vi "Analyze_Splitting_vs_Angle.vi"(11 "X,Y,Z1, Z2, ...":dbl[][](array[numeric])=array2435x8[19480 elements]) -> (3 "Intensity Graph":dbl[][](graph))   [LabVIEW 2016]
uses:
  <vilib>/gmath/NumericalOptimization/Nonlinear Curve Fit LM formula string.vi
  <vilib>/gmath/NI_Gmath.lvlib
  <vilib>/Analysis/NI_AALPro.lvlib
panel:
  out "best fit parameters 2":dbl[](array[numeric])=[10.0, 160.0, 170.0]
  in  "initial parameters 2":dbl[](array[numeric])=[10.0, 160.0, 170.0]
  in  "model description 2":T1={"model"="a*sin(3.14/180*(x-b))+c", "Parameters"=["a", "b", "c"], "x"="x"}
  in  "which fitting parameter to plot":i32=1
  in  "Enum 2":enum16{"All Phi", "Phi from cursor"}(ring)=enum."Phi from cursor"
  in  "Load New Data?":bool
  in  "STOP":bool=TRUE
  in  "2D Array Settings":T2={"x Max"=270.0, "x Min"=65.0, "x step size"=2.5, "y Max"=320.0, "y Min"=5.0, "y step size"=2.5} {"y step size" format="%#_13g"; "y Min" format="%#_13g"; "y Max" format="%#_13g"; "x step size" format="%#_13g"; "x Min" format="%#_13g"; "x Max" format="%#_13g"}
  in  "limits 2":T3={"X upper limit"=260.0, "X lower limit"=60.0, "Y upper limit"=180.0, "Y lower limit"=0.0} {"Y lower limit" format="%#_13g"; "Y upper limit" format="%#_13g"; "X lower limit" format="%#_13g"; "X upper limit" format="%#_13g"}
  in  "limits":T3={"X upper limit"=215.0, "X lower limit"=120.0, "Y upper limit"=60.0, "Y lower limit"=0.0} {"Y lower limit" format="%#_13g"; "Y upper limit" format="%#_13g"; "X lower limit" format="%#_13g"; "X upper limit" format="%#_13g"}
  in  "String":string="a-((x - b)/c)*((x - b)/c)\n\na*cos(c*(x-b))"
  out "XY Graph 5":cluster{dbl[], "Best Linear Fit":dbl[]}[](graph)=[{[5.0, 7.5, 10.0, 12.5, 15.0, 17.5, 20.0, 22.5, 25.0, 27.5, 30.0, 32.5, 35.0, 37.5, 40.0, 42.5, 45.0, 47.5, 50.0, 52.5, 55.0, 57.5, 60.0, 62.5, 65.0, 67.5, 70.0, 72.5, 75.0, 77.5, 80.0, 82.5, 85.0, 87.5, 90.0, 92.5, 95.0, 97.5, 100.0, 102.5, 105.0, 107.5, 110.0, 112.5, 115.0, 117.5, 120.0, 122.5, 125.0, 127.5, 130.0, 132.5, 135.0, 137.5, 140.0, 142.5, 145.0, 147.5, 150.0, 152.5, 155.0, 157.5, 160.0, 162.5, 165.0, 167.5, 170.0, 172.5, 175.0, 177.5, 180.0, 182.5, 185.0, 187.5, 190.0, 192.5, 195.0, 197.5, 200.0, 202.5, 205.0, 207.5, 210.0, 212.5, 215.0, 217.5, 220.0, 222.5, 225.0, 227.5, 230.0, 232.5, 235.0, 237.5, 240.0, 242.5, 245.0, 247.5, 250.0, 252.5, 255.0, 257.5, 260.0, 262.5, 265.0, 267.5, 270.0, 272.5, 275.0, 277.5, 280.0, 282.5, 285.0, 287.5, 290.0, 292.5, 295.0, 297.5, 300.0, 302.5, 305.0, 307.5, 310.0, 312.5, 315.0, 317.5, 320.0], "Best Linear Fit"=[158.21586008274636]}, {[5.0, 7.5, 10.0, 12.5, 15.0, 17.5, 20.0, 22.5, 25.0, 27.5, 30.0, 32.5, 35.0, 37.5, 40.0, 42.5, 45.0, 47.5, 50.0, 52.5, 55.0, 57.5, 60.0, 62.5, 65.0, 67.5, 70.0, 72.5, 75.0, 77.5, 80.0, 82.5, 85.0, 87.5, 90.0, 92.5, 95.0, 97.5, 100.0, 102.5, 105.0, 107.5, 110.0, 112.5, 115.0, 117.5, 120.0, 122.5, 125.0, 127.5, 130.0, 132.5, 135.0, 137.5, 140.0, 142.5, 145.0, 147.5, 150.0, 152.5, 155.0, 157.5, 160.0, 162.5, 165.0, 167.5, 170.0, 172.5, 175.0, 177.5, 180.0, 182.5, 185.0, 187.5, 190.0, 192.5, 195.0, 197.5, 200.0, 202.5, 205.0, 207.5, 210.0, 212.5, 215.0, 217.5, 220.0, 222.5, 225.0, 227.5, 230.0, 232.5, 235.0, 237.5, 240.0, 242.5, 245.0, 247.5, 250.0, 252.5, 255.0, 257.5, 260.0, 262.5, 265.0, 267.5, 270.0, 272.5, 275.0, 277.5, 280.0, 282.5, 285.0, 287.5, 290.0, 292.5, 295.0, 297.5, 300.0, 302.5, 305.0, 307.5, 310.0, 312.5, 315.0, 317.5, 320.0], "Best Linear Fit"=[0.0, 0.0, 0.0, 0.0, 0.0, 0.0, 0.0, 0.0, 0.0, 0.0, 0.0, 0.0, 0.0, 0.0, 0.0, 0.0, 0.0, 0.0, 0.0, 0.0, 0.0, 0.0, 0.0, 0.0, 0.0, 0.0, 0.0, 0.0, 0.0, 0.0, 0.0, 0.0, 0.0, 0.0, 0.0, 0.0, 0.0, 0.0, 0.0, 0.0, 0.0, 0.0, 0.0, 0.0, 0.0, 0.0, 0.0, 0.0, 0.0, 0.0, 0.0, 0.0, 0.0, 0.0, 0.0, 0.0, 0.0, 0.0, 0.0, 0.0, 0.0, 0.0, 0.0, 0.0, 0.0, 0.0, 0.0, 0.0, 0.0, 0.0, 0.0, 0.0, 0.0, 0.0, 0.0, 0.0, 0.0, 0.0, 0.0, 0.0, 0.0, 0.0, 0.0, 0.0, 0.0, 0.0, 0.0, 0.0, 0.0, 0.0, 0.0, 0.0, 0.0, 0.0, 0.0, 0.0, 0.0, 0.0, 0.0, 0.0, 0.0, 0.0, 0.0, 0.0, 0.0, 0.0, 0.0, 0.0, 0.0, 0.0, 0.0, 0.0, 0.0, 0.0, 0.0, 0.0, 0.0, 0.0, 0.0, 0.0, 0.0, 0.0, 0.0, 0.0, 0.0, 0.0, 0.0]}]
  out "best fit parameters":dbl[](array[numeric])=[50.324461350377526, 158.21586008274636, -25.837217688532053]
  in  "initial parameters":dbl[](array[numeric])=[10.0, 170.0, 10.0]
  in  "model description":T1={"model"="a*cos(3.14/180*(x-b))*cos(3.14/180*(x-b))+c", "Parameters"=["a", "b", "c"], "x"="x"}
  in  "Enum":T4(ring)
  out "XY Graph 4":cluster{"Waveform Graph":dbl[], dbl[]}[](graph)=[{"Waveform Graph"=[65.0, 67.5, 70.0, 72.5, 75.0, 77.5, 80.0, 82.5, 85.0, 87.5, 90.0, 92.5, 95.0, 97.5, 100.0, 102.5, 105.0, 107.5, 110.0, 112.5, 115.0, 117.5, 120.0, 122.5, 125.0, 127.5, 130.0, 132.5, 135.0, 137.5, 140.0, 142.5, 145.0, 147.5, 150.0, 152.5, 155.0, 157.5, 160.0, 162.5, 165.0, 167.5, 170.0, 172.5, 175.0, 177.5, 180.0, 182.5, 185.0, 187.5, 190.0, 192.5, 195.0, 197.5, 200.0, 202.5, 205.0, 207.5, 210.0, 212.5, 215.0, 217.5, 220.0, 222.5, 225.0, 227.5, 230.0, 232.5, 235.0, 237.5, 240.0, 242.5, 245.0, 247.5, 250.0, 252.5, 255.0, 257.5, 260.0, 262.5, 265.0, 267.5, 270.0], [-1.0, -1.0, -1.0, -1.0, -1.0, -1.0, -1.0, -1.0, -1.0, -1.0, -1.0, -1.0, -1.0, -1.0, -1.0, -1.0, -1.0, -1.0, -1.0, -1.0, -1.0, -1.0, -1.0, -1.0, -1.0, -1.0, -1.0, -1.0, -1.0, 18.418380709944255, 19.535911391444284, 20.466898621255627, 21.78744699669355, 22.5401738211584, 23.818559390972425, 24.547534188555957, 23.841433300349628, -1.0, -1.0, -1.0, -1.0, -1.0, -1.0, -1.0, -1.0, -1.0, -1.0, -1.0, -1.0, -1.0, -1.0, -1.0, -1.0, -1.0, -1.0, -1.0, -1.0, -1.0, -1.0, -1.0, -1.0, -1.0, -1.0, -1.0, -1.0, -1.0, -1.0, -1.0, -1.0, -1.0, -1.0, -1.0, -1.0, -1.0, -1.0, -1.0, -1.0, -1.0, -1.0, -1.0, -1.0, -1.0]}, {"Waveform Graph"=[65.0, 67.5, 70.0, 72.5, 75.0, 77.5, 80.0, 82.5, 85.0, 87.5, 90.0, 92.5, 95.0, 97.5, 100.0, 102.5, 105.0, 107.5, 110.0, 112.5, 115.0, 117.5, 120.0, 122.5, 125.0, 127.5, 130.0, 132.5, 135.0, 137.5, 140.0, 142.5, 145.0, 147.5, 150.0, 152.5, 155.0, 157.5, 160.0, 162.5, 165.0, 167.5, 170.0, 172.5, 175.0, 177.5, 180.0, 182.5, 185.0, 187.5, 190.0, 192.5, 195.0, 197.5, 200.0, 202.5, 205.0, 207.5, 210.0, 212.5, 215.0, 217.5, 220.0, 222.5, 225.0, 227.5, 230.0, 232.5, 235.0, 237.5, 240.0, 242.5, 245.0, 247.5, 250.0, 252.5, 255.0, 257.5, 260.0, 262.5, 265.0, 267.5, 270.0], [-25.683463517298065, -25.830339145701984, -25.785961294277126, -25.550667363130934, -25.126246267118493, -24.5159248349122, -23.724343275764923, -22.757519900490145, -21.62280536488183, -20.328826783456435, -18.8854221384143, -17.303565482502236, -15.59528350445201, -13.773564091338768, -11.852257583050275, -9.845971469618654, -7.76995933201971, -5.640004870811225, -3.472301904328134, -1.283331248795708, 0.910264583571923, 3.0918079158306853, 5.24471270491917, 7.3526106435886085, 9.399475606910503, 11.369745497208147, 13.24844056103829, 15.02127727867104, 16.67477696017865, 18.19636822248845, 19.57448256827774, 20.798642340034664, 21.85954038057915, 22.74911079439403, 23.460590271774894, 23.988569509557944, 24.329034337479445, 24.479396237487375, 24.438512023970258, 24.206692535276257, 23.78570027044226, 23.178735989100087, 22.390414376439924, 21.426728958247143, 20.295006532760123, 19.00385146579877, 17.563080272681777, 15.983646984299707, 14.277559864777476, 12.457790113913145, 10.53817324851875, 8.533303912450325, 6.458424915075337, 4.3293113418063705, 2.1621506177963603, -0.026580563341561003, -2.2202415100917356, -4.402154050452324, -6.55572933431181, -8.664593956720644, -10.712714443156154, -12.684519150332303, -14.565016655755544, -16.33990973592333, -17.995704066601217, -19.51981081874172, -20.90064237001925, -22.12770040429616, -23.191655729209227, -24.084419205031793, -24.799203245546956, -25.330573423347154, -25.674489787210614, -25.828337577422865, -25.790947105518118, -25.562602647296874, -25.145040281507086, -24.54143469062121, -23.756375024061345, -22.795830007381902, -21.667102562680963, -20.378774285256476, -18.940640198645482]}]
  # "Fit stuff vs theta"
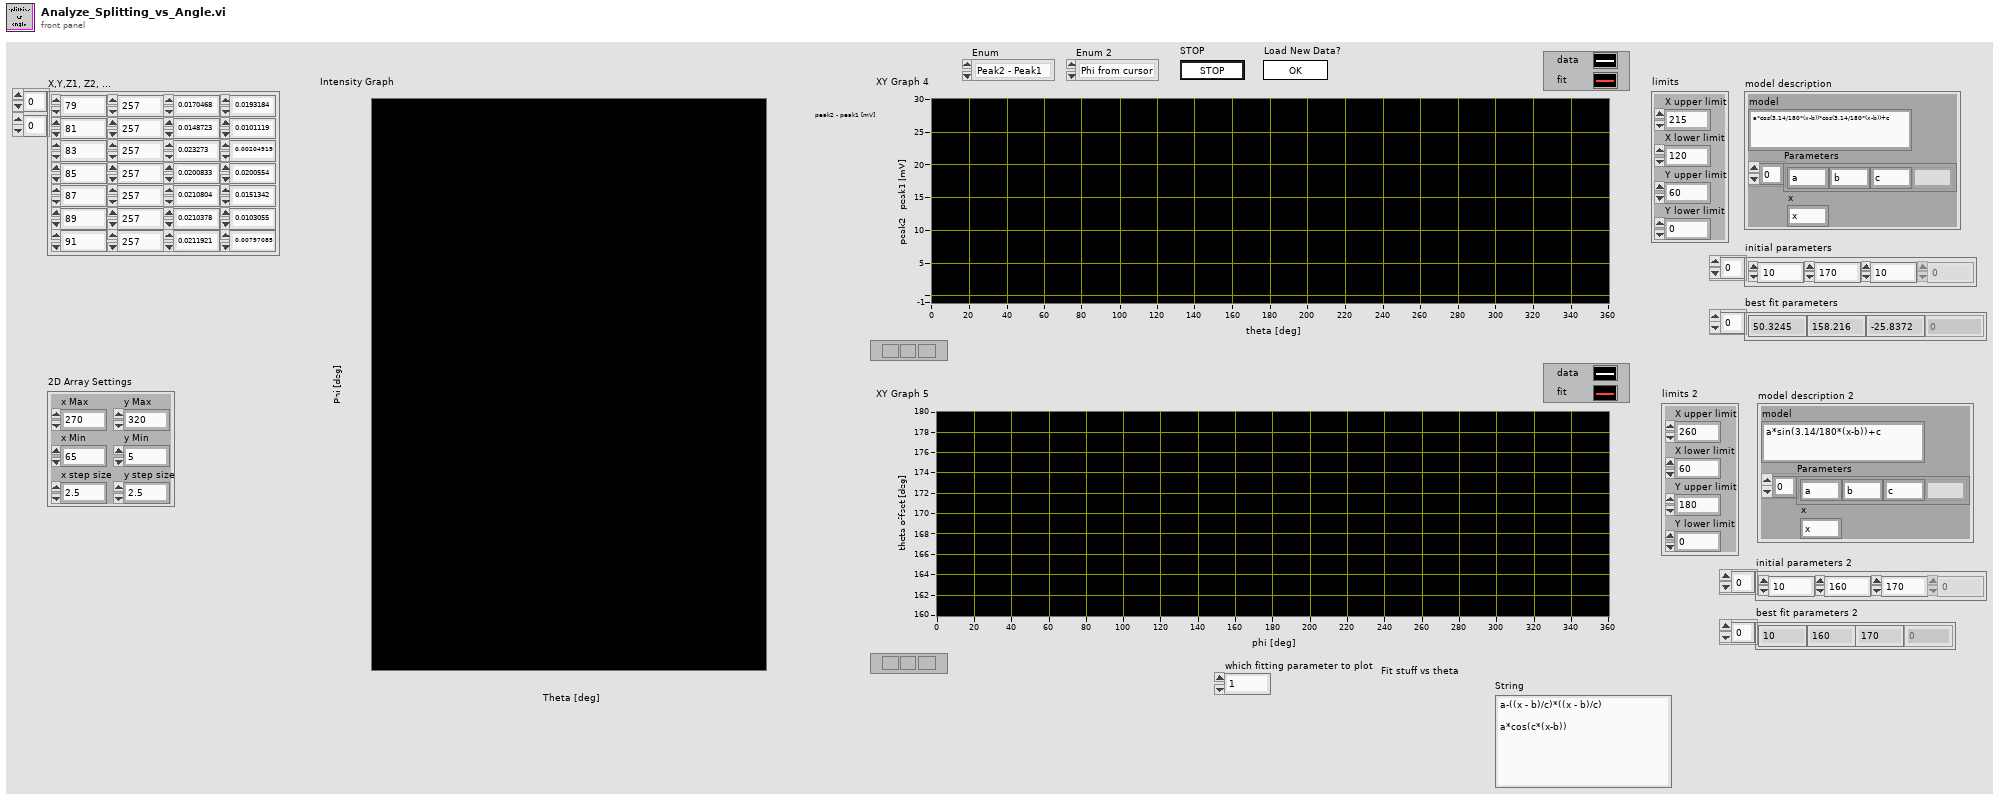
[diagram p1: front panel]
types:
  T1 = cluster{"model":string, "Parameters":string[], "x":string}
  T2 = cluster{"x Max":dbl, "x Min":dbl, "x step size":dbl, "y Max":dbl, "y Min":dbl, "y step size":dbl}
  T3 = cluster{"X upper limit":dbl, "X lower limit":dbl, "Y upper limit":dbl, "Y lower limit":dbl}
  T4 = enum16{"Peak2 - Peak1", "Peak3 - Peak2", "Peak3 - Peak1"}
  T5 = enum32{"invalid app kind", "Development System", "Run Time System", "Student Edition", "Embedded LabVIEW", "Evaluation", "Custom"}
  T6 = enum32{"Invalid", "Standard", "Closed", "Hidden", "Minimized", "Maximized"}
  T7 = cluster{"Core":cluster{"Current VI Reference":refnum<vi>, "Close Panel on Exit?":bool}, "Your Boolean data":bool, "Your string data":string, "2D array":dbl[][], "x array":dbl[], "y array":dbl[], "best fitting":dbl[][], "fitting goodness":dbl[][]}
  T8 = cluster{"Current VI Reference":refnum<vi>, "Close Panel on Exit?":bool}
  T9 = typedef "LVOffsetAndMultiplierTypeDef.ctl" = cluster{"Offset":dbl, "Multiplier":dbl}
  T10 = typedef "LVPointDoubleTypeDef.ctl" = cluster{"Cursor X":dbl, "Cursor Y":dbl}
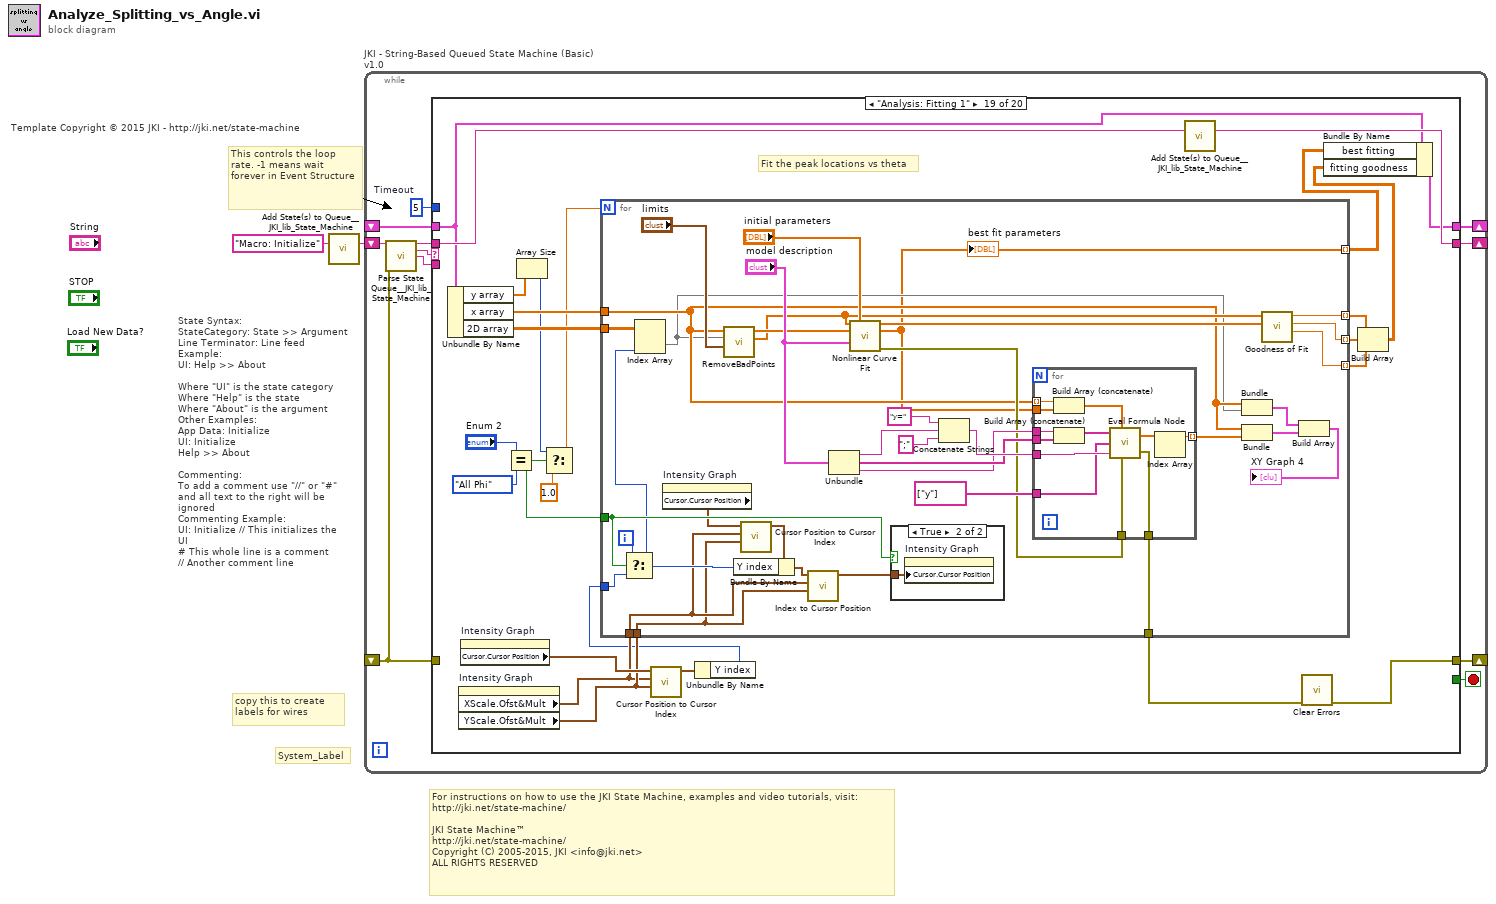
[diagram p0: block diagram]
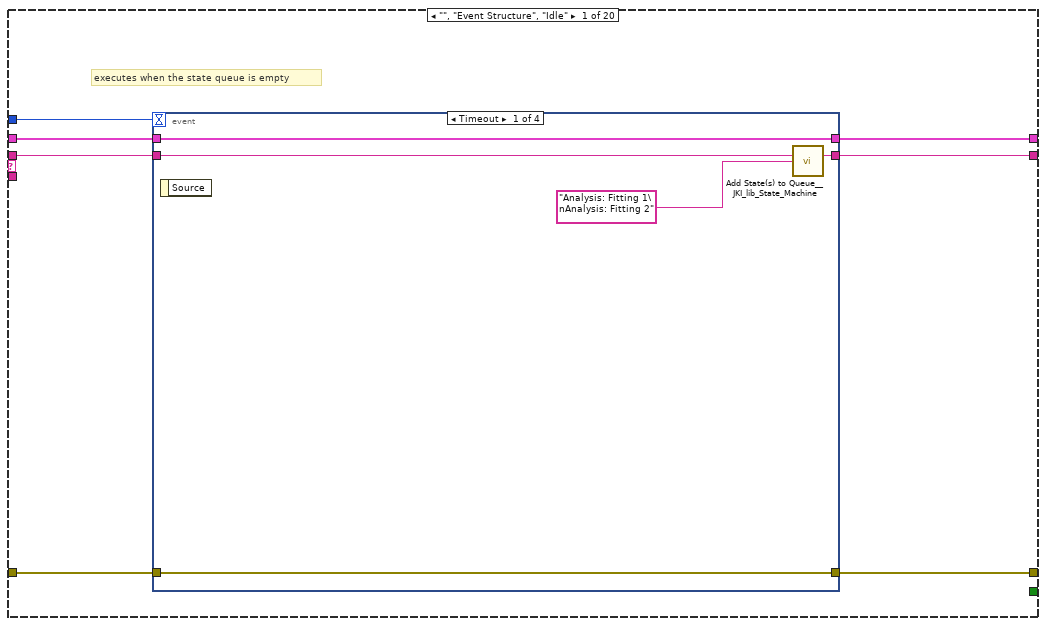
[diagram p2: hidden frame]
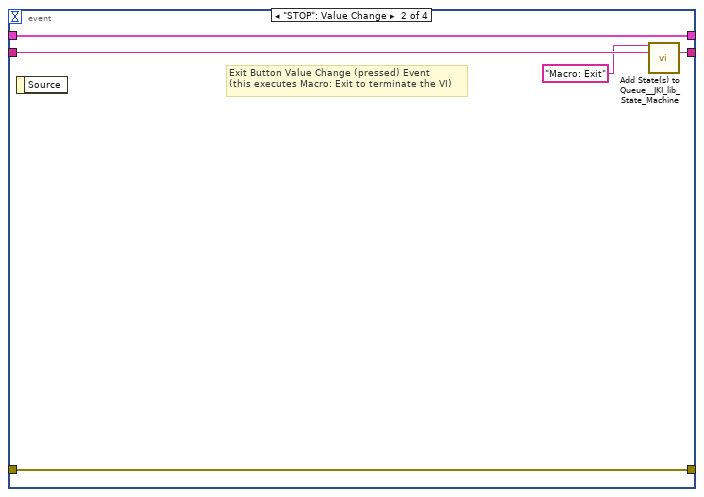
[diagram p3: hidden frame]
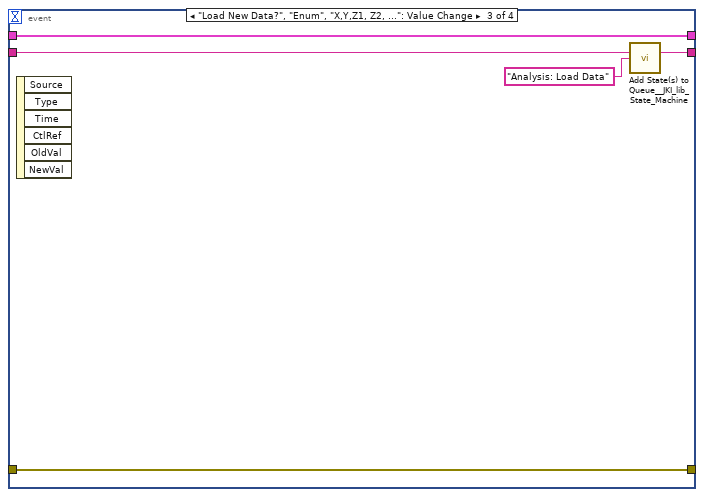
[diagram p4: hidden frame]
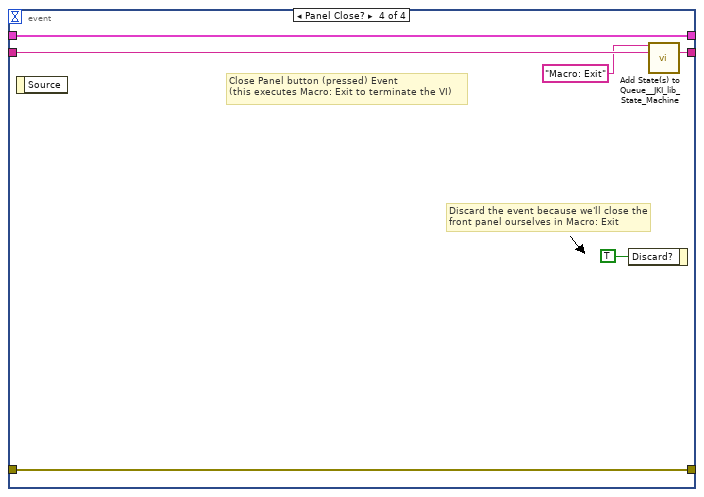
[diagram p5: hidden frame]
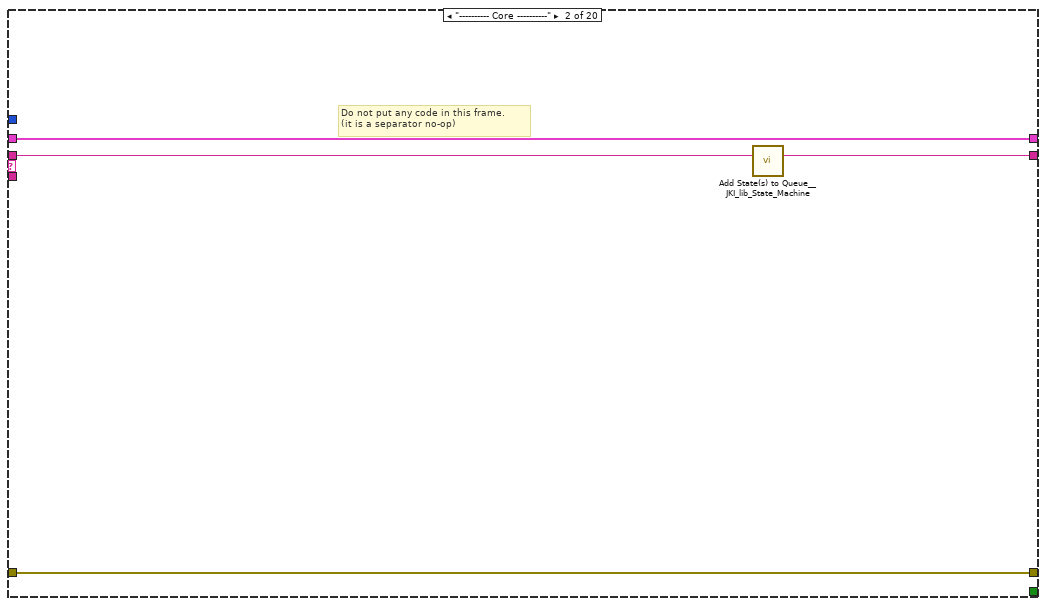
[diagram p6: hidden frame]
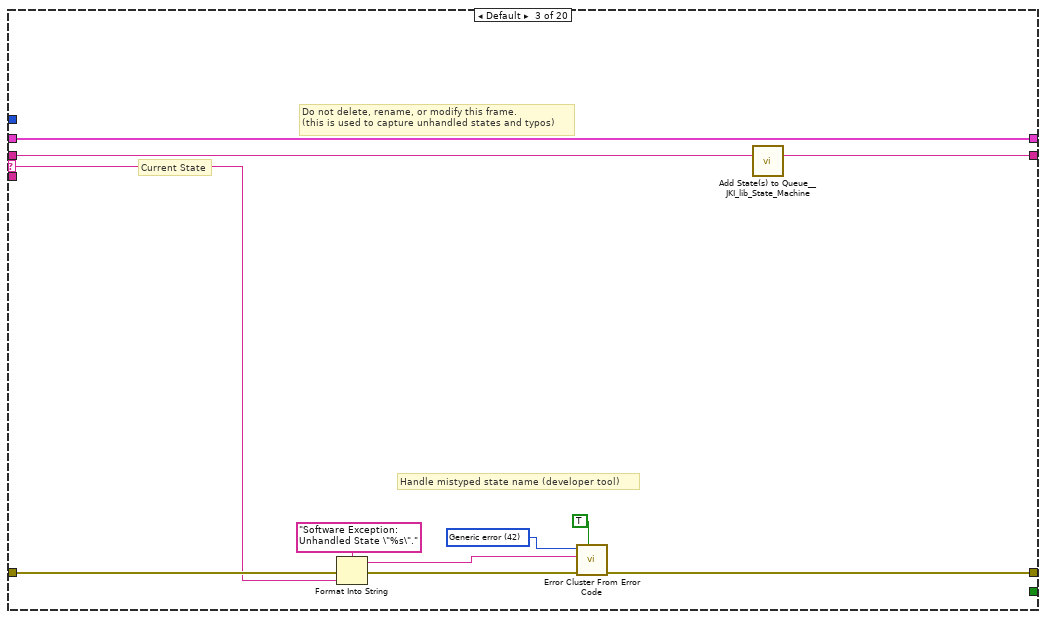
[diagram p7: hidden frame]
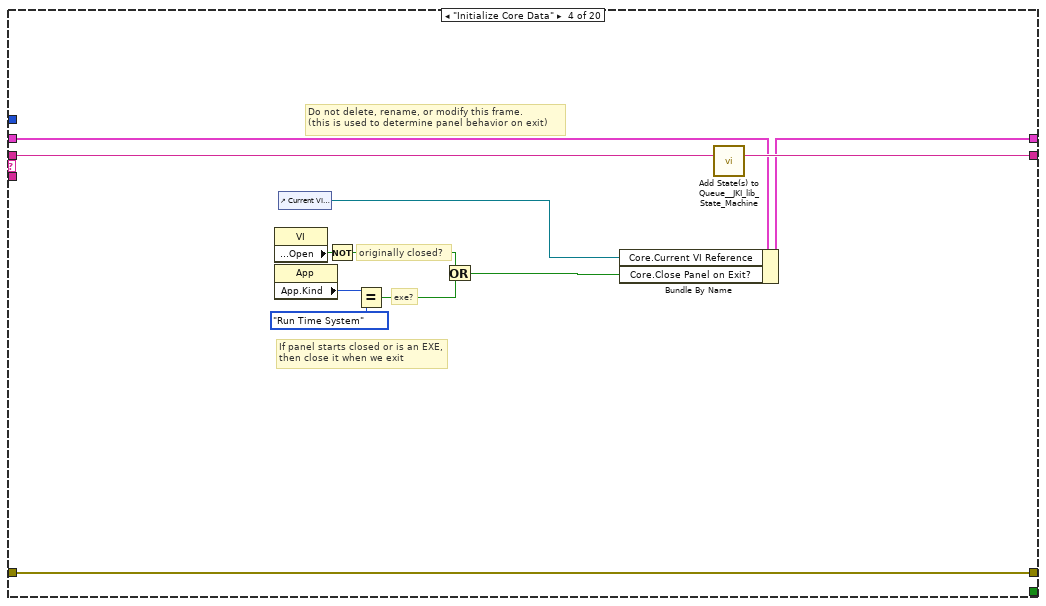
[diagram p8: hidden frame]
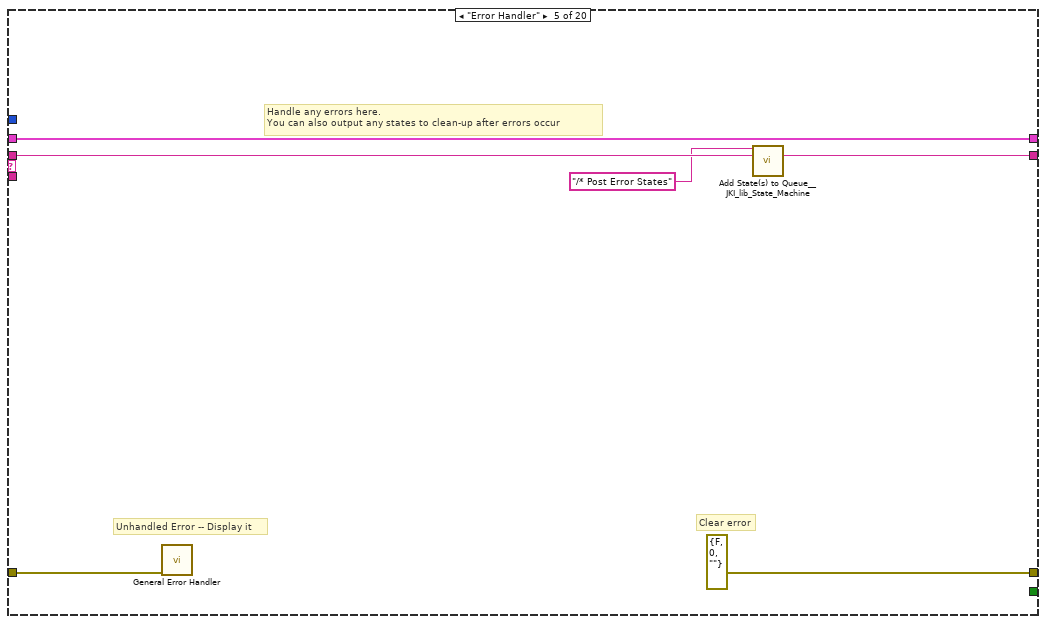
[diagram p9: hidden frame]
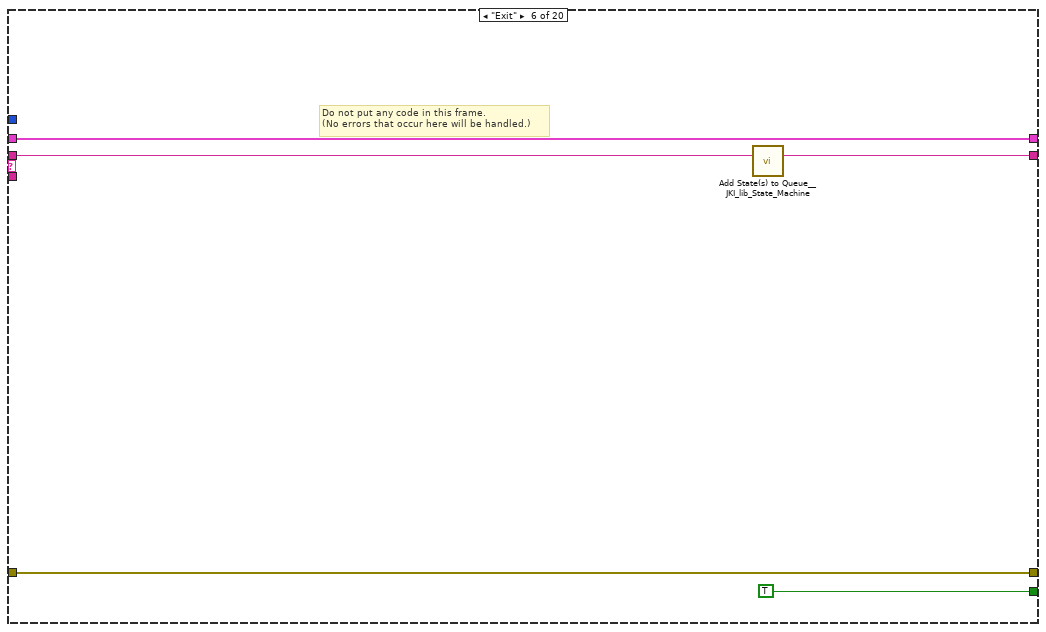
[diagram p10: hidden frame]
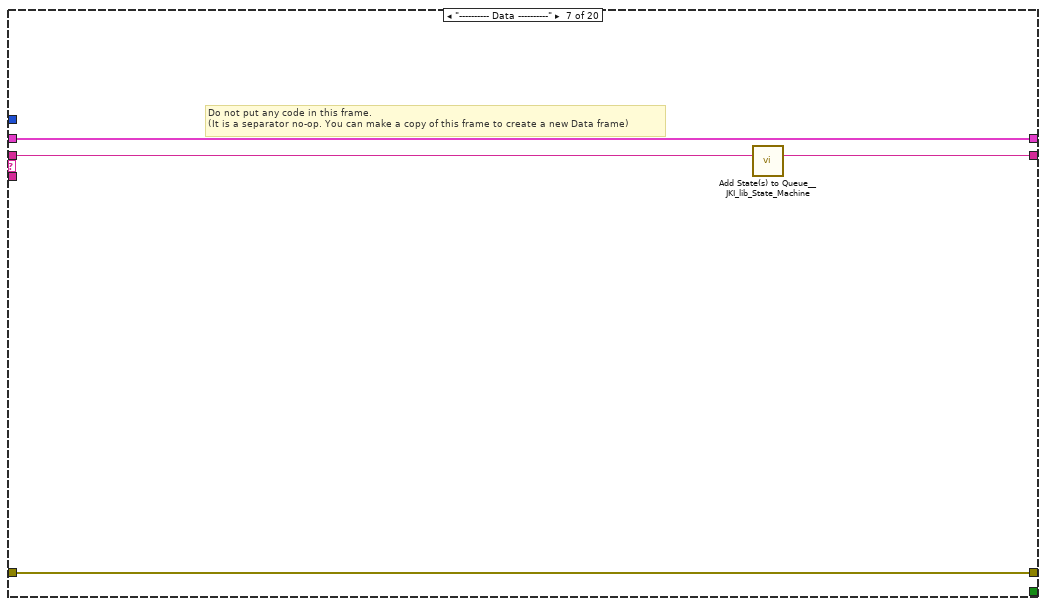
[diagram p11: hidden frame]
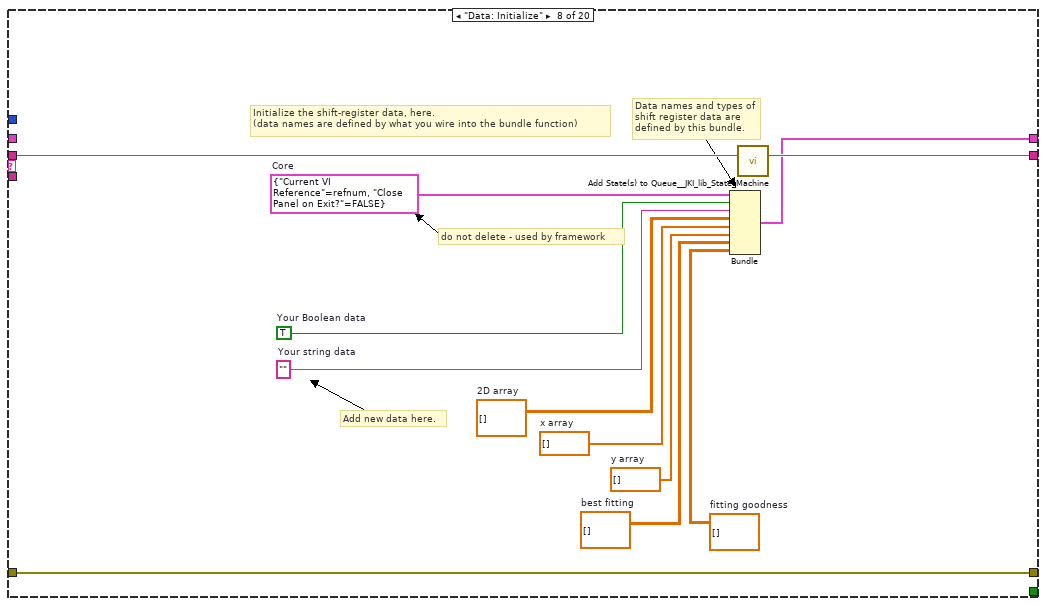
[diagram p12: hidden frame]
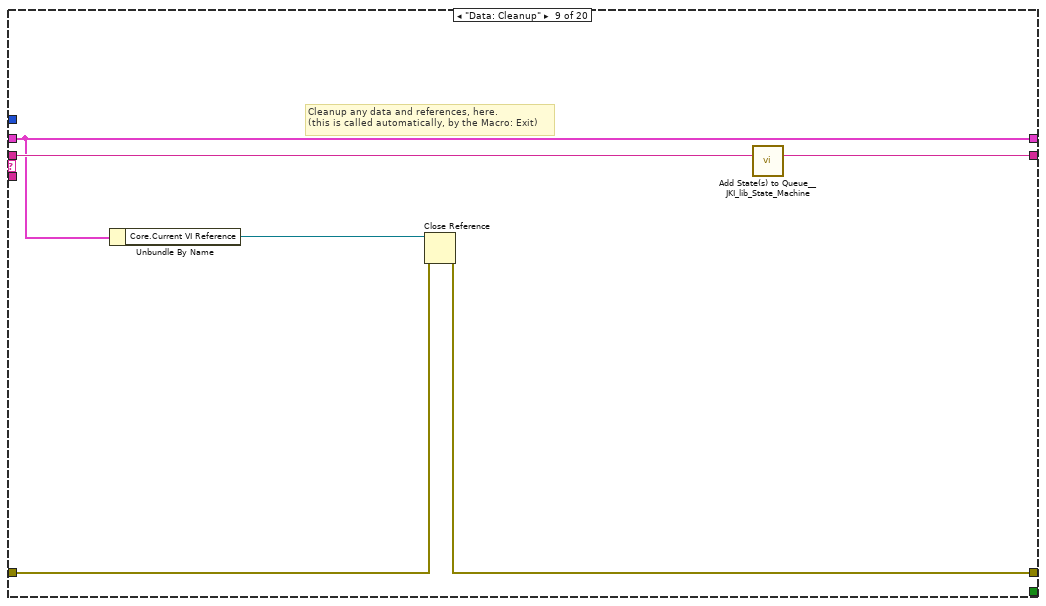
[diagram p13: hidden frame]
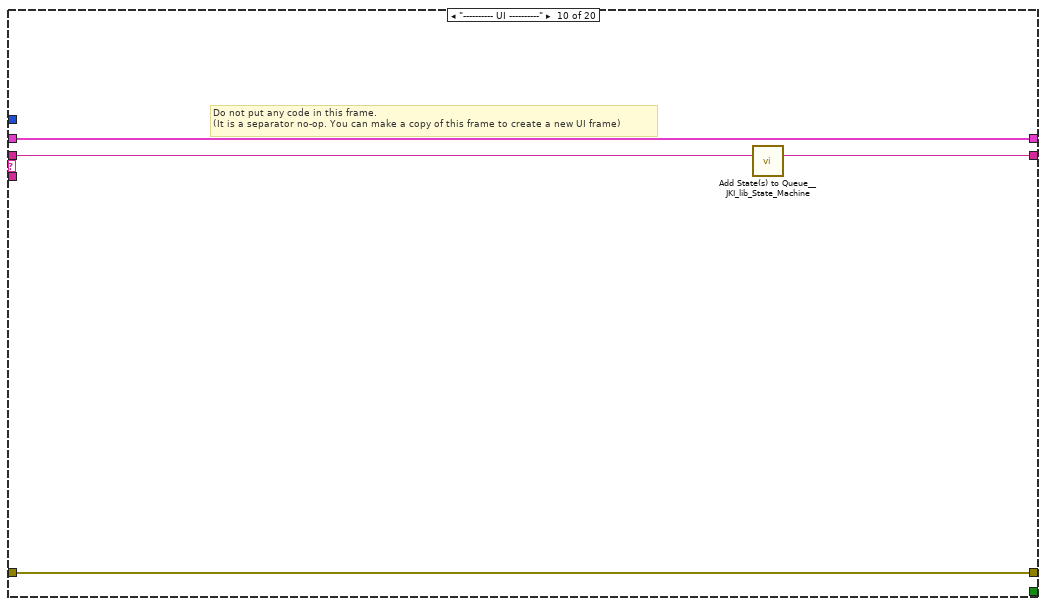
[diagram p14: hidden frame]
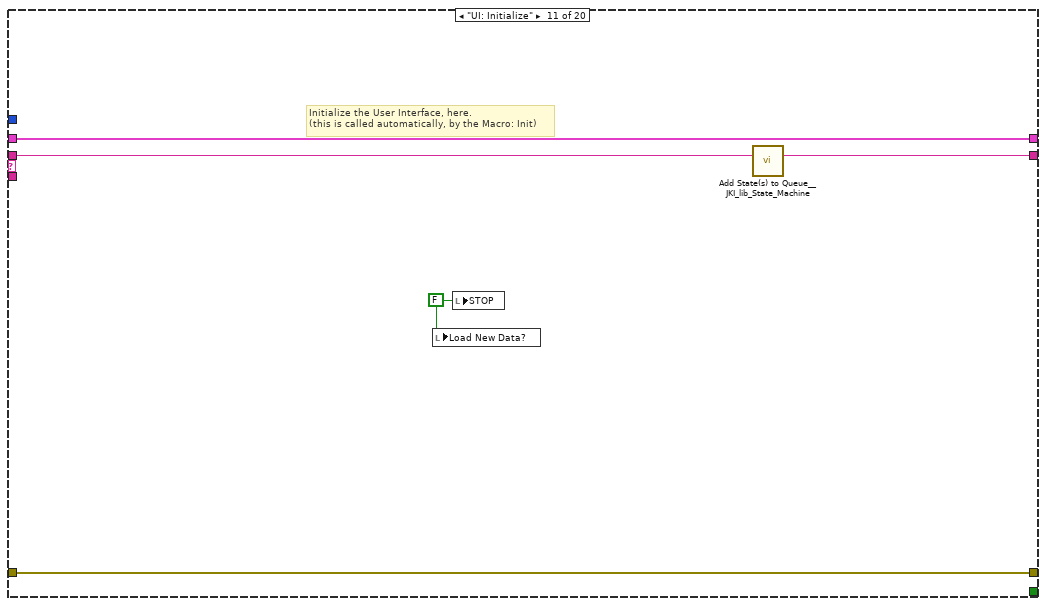
[diagram p15: hidden frame]
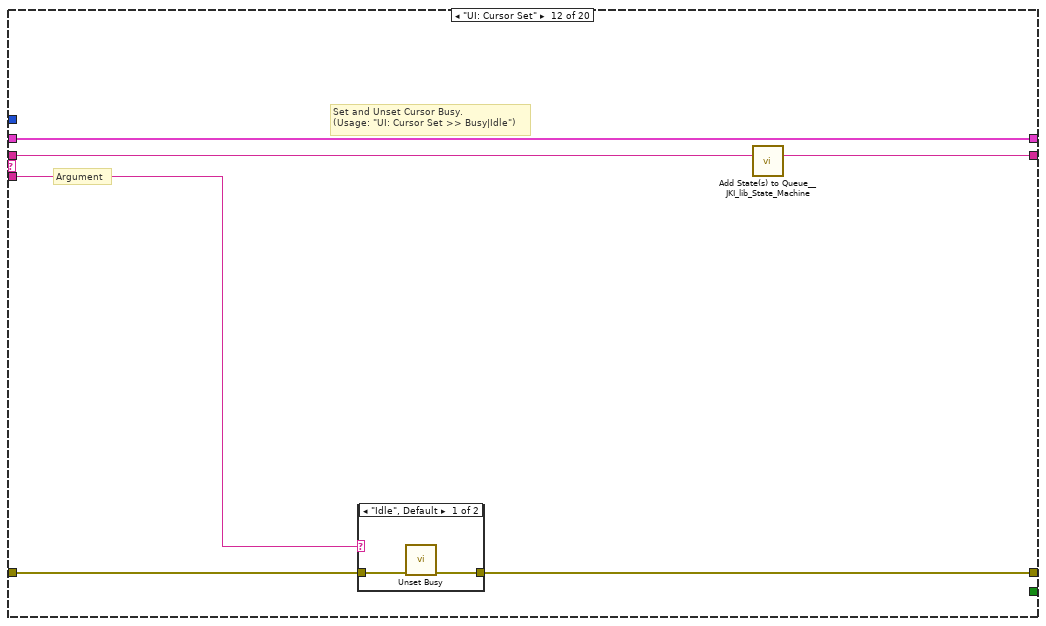
[diagram p16: hidden frame]
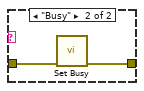
[diagram p17: hidden frame]
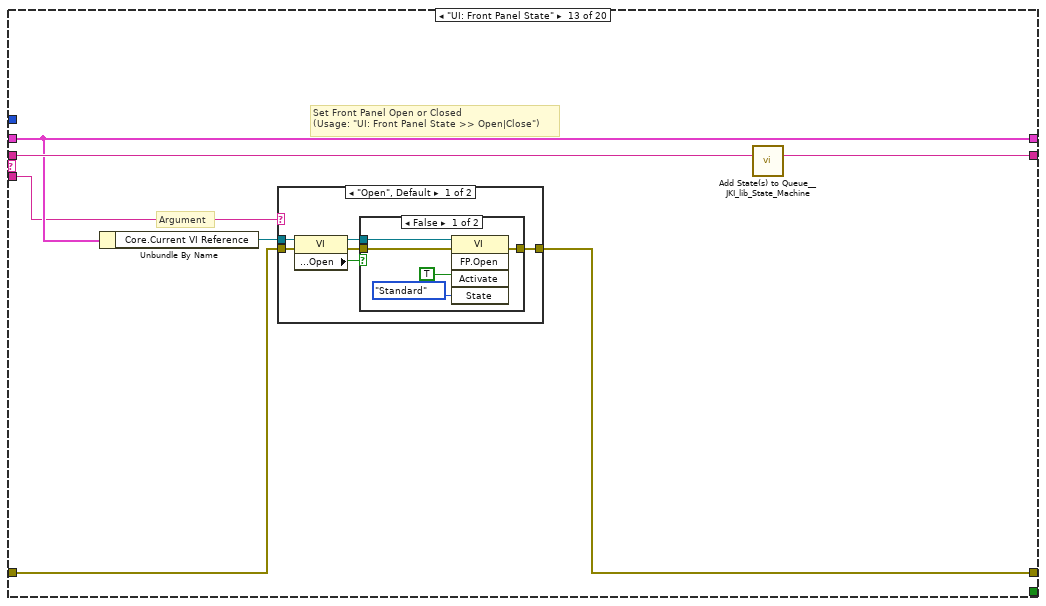
[diagram p18: hidden frame]
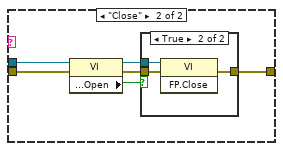
[diagram p20: hidden frame]
diagram:
  # "Template Copyright © 2015 JKI - http://jki.net/state-machine"
  # "For instructions on how to use the JKI State Machine, examples and video tutorials, visit:\nhttp://jki.net/state-machine/\n\nJKI State Machine™\nhttp://jki.net/state-machine/\nCopyright (C) 2005-2015, JKI <info@jki.net>\nALL RIGHTS RESERVED"
  # "State Syntax:\nStateCategory: State >> Argument\nLine Terminator: Line feed\nExample:\nUI: Help >> About\n\nWhere \"UI\" is the state category\nWhere \"Help\" is the state\nWhere \"About\" is the argument\nOther Examples:\nApp Data: Initialize\nUI: Initialize\nHelp >> About\n\nCommenting:\nTo add a comment use \"//\" or \"#\" and all text to the right will be ignored\nCommenting Example:\nUI: Initialize // This initializes the UI\n# This whole line is a comment\n// Another comment line"
  # "copy this to create labels for wires"
  # "This controls the loop rate. -1 means wait forever in Event Structure"
  # "System_Label"
  n1 = call <vilib>:"Add State(s) to Queue__JKI_lib_State_Machine.vi"("State(s) in (\"\")"="Macro: Initialize") -> ("States Out"=w2:string)  [unwired: 14 in]
  n2 = while "JKI - String-Based Queued State Machine (Basic) v1.0" {
    shift-right: [w6] -> _
    shift-left: _ -> [w5]
    shift-right: [w9] -> _
    shift-left: _ -> [w3]
    shift-right: [w8] -> _
    shift-left: w2 -> [w10]
    stop <- w7 stop-if-true
    w4 = 5  # Timeout
    n3 = call <vilib>:"Parse State Queue__JKI_lib_State_Machine.vi"("State Queue"=w10, "Error In (no error)"=w3) -> ("Remaining States"=w12:string, "Current State"=w13:string, "Arguments"=w11:string)  [unwired: 11 in]
    n4 = case shown="\"Analysis: Fitting 1\"" w13 {
      selector: w13 -> [_ _ w46 _ _ _ _ _ _ _ _ _ _ _ _ _ _ _ _ _]
      tunnel: w12 -> [w20 w45 w50 w68 w74 w79 w83 w95 w101 w105 w110 w116 w127 w153 w158 w168 w172 w193 w217 w295]
      tunnel: w11 -> [_ _ _ _ _ _ _ _ _ _ _ w111 w121 _ _ _ _ _ _ _]
      tunnel: w5 -> [w18 w42 w48 w59 w71 w77 w80 _ w96 w102 w108 w114 w123 w150 w155 w165 w169 w173 w208 w294]
      tunnel: [w14 w43 w52 w65 errorcluster {"status"=FALSE, "code"=0, "source"=""} ("error out") w76 w81 w92 w97 w103 w107 w112 w124 w151 w156 w166 w170 w191 w203 w277] -> w9
      tunnel: w3 -> [w17 w43 w51 w65 w70 w76 w81 w92 w98 w103 w107 w113 w125 w151 w156 w166 w170 w191 _ w276]
      tunnel: [w19 w44 w49 w67 w73 w78 w82 w94 w100 w104 w109 w115 w126 w152 w157 w167 w171 w192 w218 w295] -> w8
      tunnel: [_ _ _ _ _ TRUE _ _ _ _ _ _ _ _ _ _ _ _ _ _] -> w7
      tunnel: [w16 w42 w48 w66 w71 w77 w80 w93 w96 w102 w108 w114 w123 w150 w155 w165 w169 w174 w204 w294] -> w6
      tunnel: w4 -> [w15 _ _ _ _ _ _ _ _ _ _ _ _ _ _ _ _ _ _ _]
      frame "", "Event Structure", "Idle" {
        # "executes when the state queue is empty"
        n5 = event shown="[0] Timeout" {
          selector: _ -> [_ _ _ _]
          dyn-events: _ -> [_ _ _ _]
          timeout: w15 -> [_ _ _ _]
          tunnel: w20 -> [w25 w30 w34 w41]
          tunnel: [w24 w29 w35 w40] -> w19
          tunnel: w18 -> [w22 w27 w33 w38]
          tunnel: w17 -> [w23 w28 w32 w39]
          tunnel: [w22 w27 w33 w38] -> w16
          tunnel: [w23 w28 w32 w39] -> w14
          event Timeout {
            n6 = event-data() -> ()  [unwired: 1 in, 1 out]
            n7 = call <vilib>:"Add State(s) to Queue__JKI_lib_State_Machine.vi"("State(s) in (\"\")"=w25, "State(s) at Back (\"\")"="Analysis: Fitting 1\nAnalysis: Fitting 2" ("State(s) at Back (\"\")")) -> ("States Out"=w24:string)  [unwired: 13 in]
          }
          event "STOP": Value Change {
            # "Exit Button Value Change (pressed) Event\n(this executes Macro: Exit to terminate the VI)"
            n8 = event-data() -> ()  [unwired: 1 in, 1 out]
            n9 = call <vilib>:"Add State(s) to Queue__JKI_lib_State_Machine.vi"("State(s) in Front (\"\")"="Macro: Exit", "State(s) in (\"\")"=w30) -> ("States Out"=w29:string)  [unwired: 13 in]
          }
          event "Load New Data?", "Enum", "X,Y,Z1, Z2, ...": Value Change {
            n10 = event-data() -> ()  [unwired: 1 in, 6 out]
            n11 = call <vilib>:"Add State(s) to Queue__JKI_lib_State_Machine.vi"("State(s) in (\"\")"=w34, "State(s) at Back (\"\")"="Analysis: Load Data" ("State(s) at Back (\"\")")) -> ("States Out"=w35:string)  [unwired: 13 in]
          }
          event Panel Close? {
            # "Discard the event because we'll close the front panel ourselves in Macro: Exit"
            # "Close Panel button (pressed) Event\n(this executes Macro: Exit to terminate the VI)"
            n12 = event-data() -> ()  [unwired: 1 in, 1 out]
            n13 = event-data("Discard?"=TRUE) -> ()  [unwired: 1 in, 1 out]
            n14 = call <vilib>:"Add State(s) to Queue__JKI_lib_State_Machine.vi"("State(s) in Front (\"\")"="Macro: Exit", "State(s) in (\"\")"=w41) -> ("States Out"=w40:string)  [unwired: 13 in]
          }
        }
      }
      frame "---------- Core ----------" {
        # "Do not put any code in this frame.\n(it is a separator no-op)"
        n15 = call <vilib>:"Add State(s) to Queue__JKI_lib_State_Machine.vi"("State(s) in (\"\")"=w45) -> ("States Out"=w44:string)  [unwired: 14 in]
      }
      frame Default {
        w55 = 42 items=["No error", "Argument error", "Memory is full", "Out of zone", "End of file", "File already open", "Generic file I/O error", "File not found", "File permission error", "Disk is full", "Duplicate path", "Too many files open", "System feature not enabled", "Resource file not found", "Cannot add resource", "Resource not found", "Image not found", "Image memory error", "Pen does not exist", "Config type invalid", "Config token not found", "Config parse error", "Config memory error", "Bad external code format", "Bad external code offset", "External code not present", "Null window", "Destroy window error", "Null menu", "Print aborted", "Bad print record", "Print driver error", "Windows error during printing", "Memory error during printing", "Print dialog error", "Generic print error", "Invalid device refnum", "Device not found", "Device parameter error", "Device unit error", "Cannot open device", "Device call aborted", "Generic error", "Cancelled by user", "Object ID too low", "Object ID too high", "Object not in heap", "Unknown heap", "Unknown object (invalid DefProc)", "Unknown object (DefProc not in table)", "Message out of range", "Invalid (null) method", "Unknown message", "Manager call not supported", "Bad address", "Network operation in progress", "Network operation timed out", "Connection is busy", "Network attribute not supported", "Network error", "Address in use", "System out of memory", "Connection aborted", "Connection refused", "Not connected", "Already connected", "Connection closed", "Initialization error (interapplication manager)", "Bad occurrence", "Wait on unbound occurrence handler", "Occurrence queue overflow", "Datalog type conflict", "Unused", "Unrecognized type (interapplication manager)", "Memory corrupt", "Failed to make temporary DLL", "Old CIN version", "Drag socket not found", "Failed to load drop-object", "Failed to register OLE object", "Failed to release OLE object", "Format specifier type mismatch", "Unknown format specifier", "Too few format specifiers", "Too many format specifiers", "Scan failed", "Newer CIN version", "Error converting to variant", "Runtime menu error", "Password tampered", "Variant attribute not found", "Incompatible variant data type", "Event data is not available", "Event Store is not present", "Occurrence is not found", "Event Queue is not created", "Event info is not available", "Refnum passed is NULL", "Error retrieving Class GUID", "Error retrieving CoClass GUID", "Error retrieving TypeLib GUID.", "Bad built application magic bytes.", "Specific driver is different from the specific driver associated with the Logical Name.", "There is no session opened to the class driver.", "Max Error", "MAX - Error with config objects", "MAX - Error loading configuration", "MAX - Group not supported"]
        # "Current State"
        # "Do not delete, rename, or modify this frame.\n(this is used to capture unhandled states and typos)"
        # "Handle mistyped state name (developer tool)"
        n16 = Format Into String(format string="Software Exception: Unhandled State \"%s\"." ("message"), error in=w51, w46) -> (resulting string=w54:string, error out=w53:errorcluster)  [unwired: 1 in]
        n17 = call <vilib>:"Error Cluster From Error Code.vi"("show call chain? (False)"=TRUE, "error in (no error)"=w53, "error message (\"\")"=w54, "error code (0)"=w55) -> ("error out"=w52:errorcluster)  [unwired: 5 in]
        n18 = call <vilib>:"Add State(s) to Queue__JKI_lib_State_Machine.vi"("State(s) in (\"\")"=w50) -> ("States Out"=w49:string)  [unwired: 14 in]
      }
      frame "Initialize Core Data" {
        # "Do not delete, rename, or modify this frame.\n(this is used to determine panel behavior on exit)"
        # "originally closed?"
        # "exe?"
        # "If panel starts closed or is an EXE, then close it when we exit"
        n19 = property class="VI"() -> ("Front Panel.Open"=w64:bool)  [unwired: 2 in, 2 out]
        n20 = property class="App"() -> ("App.Kind"=w63:T5)  [unwired: 2 in, 2 out]
        n21 = control-ref of="Current VI Reference"() -> (w57:refnum<vi>)
        n22 = Not(x=w64) -> (.not. x?=w61:bool)
        n23 = Equal?(x=w63, y=T5."Run Time System" ("Application:Kind")) -> (x = y?=w60:bool)
        n24 = Or(x=w61, y=w60) -> (x .or. y?=w58:bool)
        n25 = Bundle By Name(cluster=w59, "Core.Current VI Reference"=w57, "Core.Close Panel on Exit?"=w58) -> (w66:T7)
        n26 = call <vilib>:"Add State(s) to Queue__JKI_lib_State_Machine.vi"("State(s) in (\"\")"=w68) -> ("States Out"=w67:string)  [unwired: 14 in]
      }
      frame "Error Handler" {
        # "Unhandled Error -- Display it"
        # "Handle any errors here.\nYou can also output any states to clean-up after errors occur"
        # "Clear error"
        n27 = call <vilib>:"General Error Handler.vi"("error in (no error)"=w70) -> ()  [unwired: 10 in, 5 out]
        n28 = call <vilib>:"Add State(s) to Queue__JKI_lib_State_Machine.vi"("State(s) in Front (\"\")"="/* Post Error States", "State(s) in (\"\")"=w74) -> ("States Out"=w73:string)  [unwired: 13 in]
      }
      frame "Exit" {
        # "Do not put any code in this frame.\n(No errors that occur here will be handled.)"
        n29 = call <vilib>:"Add State(s) to Queue__JKI_lib_State_Machine.vi"("State(s) in (\"\")"=w79) -> ("States Out"=w78:string)  [unwired: 14 in]
      }
      frame "---------- Data ----------" {
        # "Do not put any code in this frame.\n(It is a separator no-op. You can make a copy of this frame to create a new Data frame)"
        n30 = call <vilib>:"Add State(s) to Queue__JKI_lib_State_Machine.vi"("State(s) in (\"\")"=w83) -> ("States Out"=w82:string)  [unwired: 14 in]
      }
      frame "Data: Initialize" {
        w84 = dbl[][] []  # fitting goodness
        w85 = dbl[][] []  # best fitting
        w86 = dbl[] []  # y array
        w87 = dbl[] []  # x array
        w88 = dbl[][] []  # 2D array
        w89 = T8 {"Current VI Reference"=refnum, "Close Panel on Exit?"=FALSE}  # Core
        w91 = TRUE  # Your Boolean data
        w90 = ""  # Your string data
        # "do not delete - used by framework"
        # "Add new data here."
        # "Data names and types of shift register data are defined by this bundle."
        # "Initialize the shift-register data, here.\n(data names are defined by what you wire into the bundle function)"
        n31 = Bundle("Core"=w89, "Your Boolean data"=w91, "Your string data"=w90, "2D array"=w88, "x array"=w87, "y array"=w86, "best fitting"=w85, "fitting goodness"=w84) -> (w93:T7)  [unwired: 1 in]
        n32 = call <vilib>:"Add State(s) to Queue__JKI_lib_State_Machine.vi"("State(s) in (\"\")"=w95) -> ("States Out"=w94:string)  [unwired: 14 in]
      }
      frame "Data: Cleanup" {
        # "Cleanup any data and references, here.\n(this is called automatically, by the Macro: Exit)"
        n33 = Unbundle By Name(w96) -> ("Core.Current VI Reference"=w99:refnum<vi>)
        n34 = Close Reference(reference=w99, error in (no error)=w98) -> (error out=w97:errorcluster)
        n35 = call <vilib>:"Add State(s) to Queue__JKI_lib_State_Machine.vi"("State(s) in (\"\")"=w101) -> ("States Out"=w100:string)  [unwired: 14 in]
      }
      frame "---------- UI ----------" {
        # "Do not put any code in this frame.\n(It is a separator no-op. You can make a copy of this frame to create a new UI frame)"
        n36 = call <vilib>:"Add State(s) to Queue__JKI_lib_State_Machine.vi"("State(s) in (\"\")"=w105) -> ("States Out"=w104:string)  [unwired: 14 in]
      }
      frame "UI: Initialize" {
        w106 = FALSE ("STOP")
        # "Initialize the User Interface, here.\n(this is called automatically, by the Macro: Init)"
        n37 = local write "Load New Data?"(w106) -> ()
        n38 = local write "STOP"(w106) -> ()
        n39 = call <vilib>:"Add State(s) to Queue__JKI_lib_State_Machine.vi"("State(s) in (\"\")"=w110) -> ("States Out"=w109:string)  [unwired: 14 in]
      }
      frame "UI: Cursor Set" {
        # "Argument"
        # "Set and Unset Cursor Busy.\n(Usage: \"UI: Cursor Set >> Busy|Idle\")"
        n40 = case shown="\"Idle\", Default" w111 {
          tunnel: w113 -> [w118 w120]
          tunnel: [w117 w119] -> w112
          frame "Idle", Default {
            n41 = call <vilib>:"Unset Busy.vi"("error in (no error)"=w118) -> ("error out"=w117:errorcluster)  [unwired: 10 in]
          }
          frame "Busy" {
            n42 = call <vilib>:"Set Busy.vi"("error in (no error)"=w120) -> ("error out"=w119:errorcluster)  [unwired: 9 in, 1 out]
          }
        }
        n43 = call <vilib>:"Add State(s) to Queue__JKI_lib_State_Machine.vi"("State(s) in (\"\")"=w116) -> ("States Out"=w115:string)  [unwired: 14 in]
      }
      frame "UI: Front Panel State" {
        # "Argument"
        # "Set Front Panel Open or Closed\n(Usage: \"UI: Front Panel State >> Open|Close\")"
        n44 = Unbundle By Name(w123) -> ("Core.Current VI Reference"=w122:refnum<vi>)
        n45 = case shown="\"Open\", Default" w121 {
          tunnel: w125 -> [w131 w144]
          tunnel: [w133 w145] -> w124
          tunnel: w122 -> [w132 w142]
          frame "Open", Default {
            n46 = property class="VI"(reference=w132, error in=w131) -> (reference out=w129:refnum<vi>, error out=w130:errorcluster, "Front Panel.Open"=w128:bool)
            n47 = case shown="False" w128 {
              tunnel: [w136 w139] -> w133
              tunnel: w130 -> [w135 w139]
              tunnel: w129 -> [w134 _]
              frame False {
                n48 = invoke class="VI" method="FP.Open"(reference=w134, error in=w135, "Activate"=TRUE, "State"=T6."Standard") -> (error out=w136:errorcluster)  [unwired: 1 in, 4 out]
              }
              frame True {
              }
            }
          }
          frame "Close" {
            n49 = property class="VI"(reference=w142, error in=w144) -> (reference out=w141:refnum<vi>, error out=w143:errorcluster, "Front Panel.Open"=w140:bool)
            n50 = case shown="True" w140 {
              tunnel: [w146 w149] -> w145
              tunnel: w143 -> [w146 w148]
              tunnel: w141 -> [_ w147]
              frame False {
              }
              frame True {
                n51 = invoke class="VI" method="FP.Close"(reference=w147, error in=w148) -> (error out=w149:errorcluster)  [unwired: 1 in, 2 out]
              }
            }
          }
        }
        n52 = call <vilib>:"Add State(s) to Queue__JKI_lib_State_Machine.vi"("State(s) in (\"\")"=w127) -> ("States Out"=w126:string)  [unwired: 14 in]
      }
      frame "---------- Macro ----------" {
        # "Do not put any code in this frame.\n(It is a separator no-op. You can make a copy of this frame to create a new Macro frame)"
        n53 = call <vilib>:"Add State(s) to Queue__JKI_lib_State_Machine.vi"("State(s) in (\"\")"=w153) -> ("States Out"=w152:string)  [unwired: 14 in]
      }
      frame "Macro: Initialize" {
        w154 = "Data: Initialize\nInitialize Core Data\nUI: Initialize\nUI: Front Panel State >> Open\nAnalysis: Load Data"  # Data: Initialize Initialize Core Data UI: Initialize UI: Front Panel State >> Open Analysis: Load Data
        # "Initialization Macro\n(This is called once, when the VI starts)"
        n54 = call <vilib>:"Add State(s) to Queue__JKI_lib_State_Machine.vi"("State(s) in Front (\"\")"=w154, "State(s) in (\"\")"=w158) -> ("States Out"=w157:string)  [unwired: 13 in]
      }
      frame "Macro: Exit" {
        # "Exit Macro\n(This is called once, when the VI exits)"
        n55 = Unbundle By Name(w165) -> ("Core.Close Panel on Exit?"=w164:bool)
        n56 = Select(t="UI: Front Panel State >> Close", s=w164, f="") -> (s? t:f=w161:string)
        n57 = call <vilib>:"Add State(s) to Queue__JKI_lib_State_Machine.vi"("State(s) in (\"\")"=w161, "State(s) at Back (\"\")"="Data: Cleanup\nExit") -> ("States Out"=w159:string)  [unwired: 13 in]
        n58 = call <vilib>:"Add State(s) to Queue__JKI_lib_State_Machine.vi"("State(s) in Front (\"\")"=w159, "State(s) in (\"\")"=w168) -> ("States Out"=w167:string)  [unwired: 13 in]
      }
      frame "---------- Analysis ----------" {
        # "Template Separator\n(You can make a copy of, or modify, this frame)"
        n59 = call <vilib>:"Add State(s) to Queue__JKI_lib_State_Machine.vi"("State(s) in (\"\")"=w172) -> ("States Out"=w171:string)  [unwired: 14 in]
      }
      frame "Analysis: Load Data" {
        # "convert to mV"
        # "Your code here.\n(You can make a copy of, or modify, this frame)"
        n60 = Index Array(array="X,Y,Z1, Z2, ...", index (col) #1=0 ("disabled index (col)")) -> (element #1=w188:dbl[], element #2=w189:dbl[], element #3=w182:dbl[], element #4=w184:dbl[], element #5=w185:dbl[])  [unwired: 9 in]
        n61 = case shown="\"Peak2 - Peak1\", Default" "Enum" {
          tunnel: w182 -> [w194 _ _]
          tunnel: [w194 w195 w196] -> w183
          tunnel: w184 -> [_ w195 _]
          tunnel: w185 -> [_ _ w196]
          frame "Peak2 - Peak1", Default {
          }
          frame "Peak3 - Peak2" {
          }
          frame "Peak3 - Peak1" {
          }
        }
        n62 = control-ref of="Intensity Graph"() -> (w190:refnum<vi>)
        n63 = Multiply(x=w183, y=1000.0) -> (x*y=w187:dbl[])
        n64 = call "XYZ to 2D Array.vi"("IntensityGraph in"=w190, "2D Array Settings"="2D Array Settings", "Z"=w187, "Y"=w189, "X"=w188) -> ("Y Array"=w176:dbl[], "X Array"=w177:dbl[], "2D Array out"=w175:dbl[][])  [unwired: 4 in]
        "Intensity Graph" <- w175
        n65 = Bundle By Name(cluster=w173, "2D array"=w175, "x array"=w177, "y array"=w176) -> (w174:T7)
        n66 = call <vilib>:"Add State(s) to Queue__JKI_lib_State_Machine.vi"("State(s) in (\"\")"=w193) -> ("States Out"=w192:string)  [unwired: 14 in]
      }
      frame "Analysis: Fitting 1" {
        # "Fit the peak locations vs theta"
        n67 = Unbundle By Name(w208) -> ("y array"=w213:dbl[], "x array"=w220:dbl[], "2D array"=w219:dbl[][])
        n68 = property on="Intensity Graph" class="IntGraph (strict)"() -> ("XScale.Ofst&Mult"=w198:T9, "YScale.Ofst&Mult"=w199:T9)  [unwired: 2 in, 2 out]
        n69 = property on="Intensity Graph" class="IntGraph (strict)"() -> ("Cursor.Cursor Position"=w200:T10)  [unwired: 2 in, 2 out]
        n70 = Equal?(x="Enum 2", y=enum16{"All Phi", "Phi from cursor"}."All Phi" ("Enum 2")) -> (x = y?=w210:bool)
        n71 = Array Size(array=w213) -> (size(s)=w211:i32)
        n72 = Select(t=w211, s=w210, f=1.0) -> (s? t:f=w212:dbl)
        n73 = call "Cursor Position to Cursor Index.vi"("YScale.Ofst&Mult"=w199, "XScale.Ofst&Mult"=w198, "Cursor Position"=w200) -> ("Index"=w209:cluster{"X index":i32, "Y index":i32})  [unwired: 8 in]
        n74 = Unbundle By Name(w209) -> ("Y index"=w197:i32)
        n75 = for {
          N: w212 -> [_]
          tunnel: w219 -> [w235]
          tunnel: w220 -> [w236]
          tunnel: [w249] -> w206 mode=indexing
          tunnel: [w248] -> w207 mode=indexing
          tunnel: [w247] -> w205 mode=indexing
          tunnel: [w237] -> w221
          tunnel: w210 -> [w229]
          tunnel: w197 -> [w228]
          tunnel: [w232] -> w201 mode=indexing
          tunnel: w199 -> [w223]
          tunnel: w198 -> [w224]
          i -> [w230]
          n76 = Select(t=w230, s=w229, f=w228) -> (s? t:f=w227:i32)
          n77 = Index Array(array=w235, index (col)=w227) -> (element=w234:dbl[])  [unwired: 1 in]
          n78 = property on="Intensity Graph" class="IntGraph (strict)"() -> ("Cursor.Cursor Position"=w226:T10)  [unwired: 2 in, 2 out]
          n79 = call "RemoveBadPoints.vi"("limits"="limits", "Y Array"=w234, "X Array"=w236) -> ("Y Array"=w245:dbl[], "X Array"=w246:dbl[])  [unwired: 7 in]
          n80 = call "Cursor Position to Cursor Index.vi"("YScale.Ofst&Mult"=w223, "XScale.Ofst&Mult"=w224, "Cursor Position"=w226) -> ("Index"=w225:cluster{"X index":i32, "Y index":i32})  [unwired: 8 in]
          n81 = Bundle By Name(cluster=w225, "Y index"=w227) -> (w222:cluster{"X index":i32, "Y index":i32})
          n82 = call "Index to Cursor Position.vi"("YScale.Ofst&Mult"=w223, "XScale.Ofst&Mult"=w224, "Index"=w222) -> ("Cursor Position"=w231:T10)  [unwired: 8 in]
          n83 = Unbundle("model description") -> ("model"=w239:string, "Parameters"=w242:string[], "x"=w241:string)
          n84 = call-poly <vilib>:"Nonlinear Curve Fit.vi"("Y"=w245, "initial parameters"="initial parameters", "X"=w246, "model description"="model description") -> ("best nonlinear fit"=w250:dbl[], "best fit parameters"=w232:dbl[], "error out"=w240:errorcluster)  [unwired: 7 in, 2 out]
          "best fit parameters" <- w232
          n85 = case shown="True" w229 {
            tunnel: w231 -> [_ w258]
            frame False {
            }
            frame True {
              n86 = property on="Intensity Graph" class="IntGraph (strict)"("Cursor.Cursor Position"=w258) -> ()  [unwired: 2 in, 2 out]
            }
          }
          n87 = Concatenate Strings("y=" ("string"), w239, ";" ("string")) -> (w252:string)
          n88 = for {
            tunnel: w252 -> [w270]
            tunnel: w241 -> [w269]
            tunnel: w242 -> [w268]
            tunnel: w236 -> [w263] mode=indexing
            tunnel: [w265] -> w256 mode=indexing
            tunnel: w232 -> [w262]
            tunnel: string[] ["y"] ("Variables Output") -> [w259]
            tunnel: w240 -> [w261]
            tunnel: [w260] -> w237
            n89 = Build Array (concatenate)(w263, w262) -> (w266:dbl[])
            n90 = Build Array (concatenate)(w269, w268) -> (w267:string[])
            n91 = call <vilib>:"Eval Formula Node.vi"("Variables Input"=w267, "Input Values"=w266, "Variables Output"=w259, "formula"=w270, "error in (no error)"=w261) -> ("Output Values"=w264:dbl[], "error out"=w260:errorcluster)
            n92 = Index Array(array=w264) -> (element=w265:dbl)  [unwired: 1 in]
          }
          n93 = Bundle("x array"=w236, "2D array"=w234) -> (w255:cluster{"x array":dbl[], "2D array":dbl[]})  [unwired: 1 in]
          n94 = Bundle("x array"=w236, w256) -> (w243:cluster{"x array":dbl[], dbl[]})  [unwired: 1 in]
          n95 = call <vilib>:"Goodness of Fit.vi"("Best Fit"=w250, "Y"=w245) -> ("RMSE"=w247:dbl, "R-square"=w248:dbl, "SSE"=w249:dbl)  [unwired: 6 in, 1 out]
          n96 = Build Array(w255, w243) -> (→"XY Graph 4":cluster{"x array":dbl[], "2D array":dbl[]}[])
        }
        n97 = call <vilib>:"Add State(s) to Queue__JKI_lib_State_Machine.vi"("State(s) in (\"\")"=w217) -> ("States Out"=w218:string)  [unwired: 14 in]
        n98 = call <vilib>:"Clear Errors.vi"("error in (no error)"=w221) -> ("error out"=w203:errorcluster)  [unwired: 5 in, 1 out]
        n99 = Build Array(w206, w207, w205) -> (w202:dbl[][])
        n100 = Bundle By Name(cluster=w208, "best fitting"=w201, "fitting goodness"=w202) -> (w204:T7)
      }
      frame "Analysis: Fitting 2" {
        # "Fit the fit vs phi"
        n101 = Unbundle By Name(w294) -> ("y array"=w271:dbl[], "best fitting"=w293:dbl[][])  [unwired: 1 out]
        n102 = Index Array(array=w293, index (col)="which fitting parameter to plot") -> (element=w291:dbl[])  [unwired: 1 in]
        n103 = call "RemoveBadPoints.vi"("limits"="limits 2", "Y Array"=w291, "X Array"=w271) -> ("Y Array"=w287:dbl[], "X Array"=w288:dbl[])  [unwired: 7 in]
        n104 = Unbundle("model description 2") -> ("model"=w280:string, "Parameters"=w282:string[], "x"=w281:string)
        n105 = call-poly <vilib>:"Nonlinear Curve Fit.vi"("Y"=w287, "initial parameters"="initial parameters 2", "X"=w288, "model description"="model description 2", "error in (no error)"=w276) -> ("best fit parameters"=w279:dbl[], "error out"=w272:errorcluster)  [unwired: 6 in, 3 out]
        "best fit parameters 2" <- w279
        n106 = Concatenate Strings("y=" ("string"), w280, ";" ("string")) -> (w284:string)
        n107 = for {
          tunnel: w284 -> [w309]
          tunnel: w281 -> [w308]
          tunnel: w282 -> [w307]
          tunnel: w271 -> [w302] mode=indexing
          tunnel: [w304] -> w275 mode=indexing
          tunnel: w279 -> [w301]
          tunnel: string[] ["y"] ("Variables Output") -> [w298]
          tunnel: w272 -> [w300]
          tunnel: [w299] -> w274
          n108 = Build Array (concatenate)(w302, w301) -> (w305:dbl[])
          n109 = Build Array (concatenate)(w308, w307) -> (w306:string[])
          n110 = call <vilib>:"Eval Formula Node.vi"("Variables Input"=w306, "Input Values"=w305, "Variables Output"=w298, "formula"=w309, "error in (no error)"=w300) -> ("Output Values"=w303:dbl[], "error out"=w299:errorcluster)
          n111 = Index Array(array=w303) -> (element=w304:dbl)  [unwired: 1 in]
        }
        n112 = call <vilib>:"Clear Errors.vi"("error in (no error)"=w274) -> ("error out"=w277:errorcluster)  [unwired: 5 in, 1 out]
        n113 = Bundle("y array"=w271, w275) -> (w292:cluster{"y array":dbl[], dbl[]})  [unwired: 1 in]
        n114 = Bundle("y array"=w271, "best fitting"=w291) -> (w290:cluster{"y array":dbl[], "best fitting":dbl[]})  [unwired: 1 in]
        n115 = Build Array(w290, w292) -> (→"XY Graph 5":cluster{"y array":dbl[], "best fitting":dbl[]}[])
      }
    }
  }
